vi "等分取数据.vi"(0 "Max":dbl, 1 "MIN":dbl, 3 "num":i32) -> (7 "数据点":dbl[](array[numeric]))   [LabVIEW 2010]
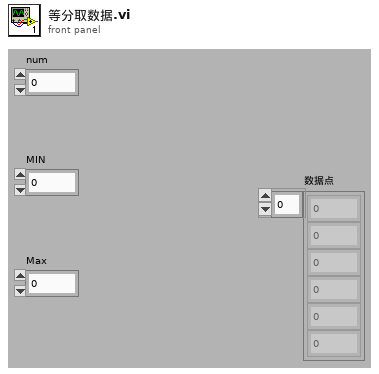
[diagram p1: front panel]
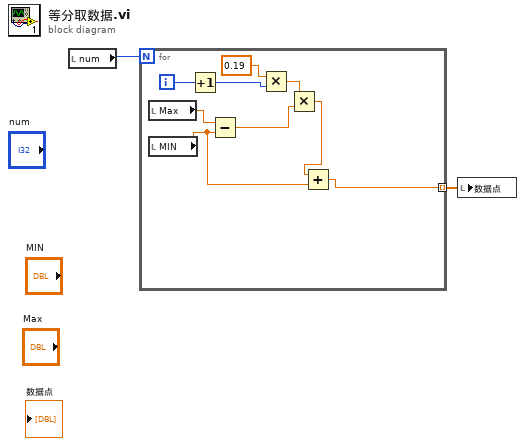
[diagram p0: block diagram]
diagram:
  n1 = local read "num"() -> (w2:i32)
  n2 = for {
    N: w2 -> [_]
    tunnel: [w3] -> w1 mode=indexing
    i -> [w9]
    n3 = local read "Max"() -> (w11:dbl)
    n4 = local read "MIN"() -> (w10:dbl)
    n5 = Increment(x=w9) -> (x+1=w7:i32)
    n6 = Subtract(x=w11, y=w10) -> (x-y=w5:dbl)
    n7 = Multiply(x=0.19, y=w7) -> (x*y=w6:dbl)
    n8 = Multiply(x=w6, y=w5) -> (x*y=w4:dbl)
    n9 = Add(x=w4, y=w10) -> (x+y=w3:dbl)
  }
  n10 = local write "数据点"(w1) -> ()
